vi "DAQ getLimits.vi"(3 "Amplitud":dbl, 5 "DAQ Device IN":T2) -> (2 "Limites":T1)   [LabVIEW 2010]
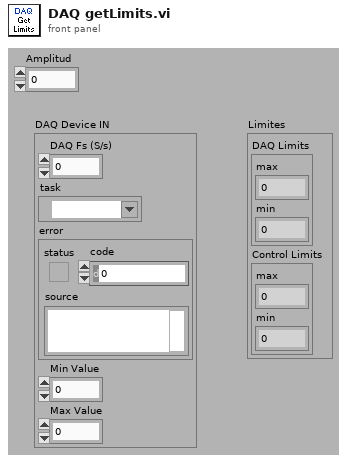
[diagram p1: front panel]
types:
  T1 = cluster{"DAQ Limits":cluster{"max":dbl, "min":dbl}, "Control Limits":cluster{"max":dbl, "min":dbl}}
  T2 = cluster{"DAQ Fs (S/s)":dbl, "task":refnum<k21>, "error":errorcluster, "Min Value":dbl, "Max Value":dbl}
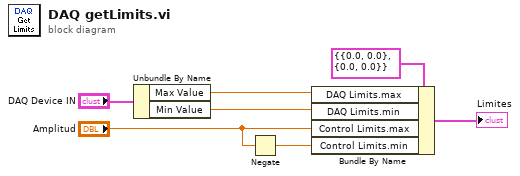
[diagram p0: block diagram]
diagram:
  n1 = Unbundle By Name("DAQ Device IN") -> ("Max Value"=w2:dbl, "Min Value"=w3:dbl)
  n2 = Negate(x="Amplitud") -> (-x=w4:dbl)
  n3 = Bundle By Name(cluster=T1 {"DAQ Limits"={"max"=0.0, "min"=0.0}, "Control Limits"={"max"=0.0, "min"=0.0}} ("Limites"), "DAQ Limits.max"=w2, "DAQ Limits.min"=w3, "Control Limits.max"="Amplitud", "Control Limits.min"=w4) -> (→"Limites":T1)
